vi "Company Header 일부.vi"() -> ()   [LabVIEW 2014]
panel:
  out "데이터 개수":string
  in  "데이터 개수 (byte)":u16
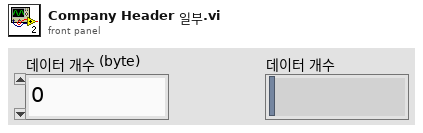
[diagram p1: front panel]
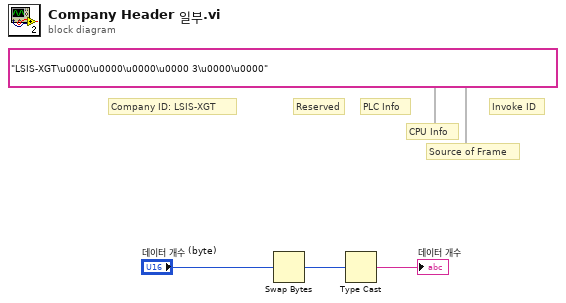
[diagram p0: block diagram]
diagram:
  (unwired) "LSIS-XGT\u0000\u0000\u0000\u0000 3\u0000\u0000"
  # "Invoke ID"
  # "Source of Frame"
  # "CPU Info"
  # "PLC Info"
  # "Reserved"
  # "Company ID: LSIS-XGT"
  n1 = Swap Bytes(anything="데이터 개수 (byte)") -> (byte swapped=w2:u16)
  n2 = Type Cast(x=w2) -> (*(type *) &x=→"데이터 개수":string)  [unwired: 1 in]
